vi "svx_Orbit Manage Grid.vi"(4 "Minor Color":u32, 6 "Major Color":u32, 7 "Axis":enum16{"X-Scale", "Y-Scale", "Z-Scale"}(ring), 10 "Grid Style":u16, 11 "Orbit Plot":refnum<vi>) -> (1 "Minor Disabled":u8, 2 "Major Disabled":u8, 3 "Orbit Plot out":refnum<vi>)   [LabVIEW 2017, in "SVX Orbit.xctl"]
uses:
  <vilib>/addons/_XControls/Orbit Plot/SVX Orbit.xctl
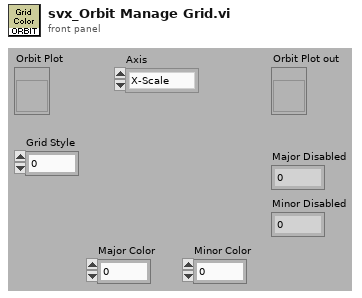
[diagram p1: front panel]
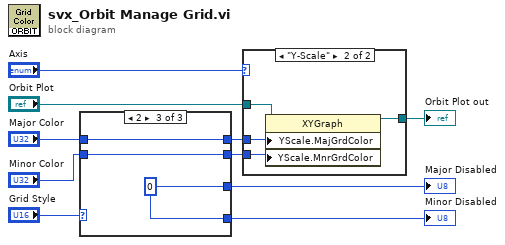
[diagram p0: block diagram]
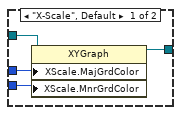
[diagram p2: hidden frame]
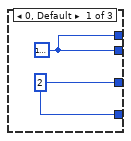
[diagram p3: hidden frame]
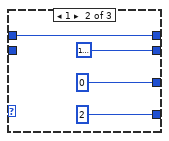
[diagram p4: hidden frame]
diagram:
  n1 = case shown="2" "Grid Style" {
    tunnel: [w12 u8 0 ("Disabled") w19] -> w7
    tunnel: [w12 u8 2 ("Disabled") w19] -> w6
    tunnel: [w11 w13 w18] -> w10
    tunnel: [w11 u32 16777216 w17] -> w5
    tunnel: "Major Color" -> [_ w13 w18]
    tunnel: "Minor Color" -> [_ _ w17]
    frame 0, Default {
      w11 = u32 16777216
      w12 = u8 2 ("Disabled")
    }
    frame 1 {
    }
    frame 2 {
      w19 = u8 0 ("Disabled")
    }
  }
  "Major Disabled" <- w7
  "Minor Disabled" <- w6
  n2 = case shown="\"Y-Scale\"" "Axis" {
    tunnel: w10 -> [w23 w27]
    tunnel: "Orbit Plot" -> [w22 w26]
    tunnel: w5 -> [w21 w25]
    tunnel: [w20 w24] -> w1
    frame "X-Scale", Default {
      n3 = property class="XYGraph"(reference=w22, "XScale.MajGrdColor"=w23, "XScale.MnrGrdColor"=w21) -> (reference out=w20:refnum<vi>)  [unwired: 1 in, 1 out]
    }
    frame "Y-Scale" {
      n4 = property class="XYGraph"(reference=w26, "YScale.MajGrdColor"=w27, "YScale.MnrGrdColor"=w25) -> (reference out=w24:refnum<vi>)  [unwired: 1 in, 1 out]
    }
  }
  "Orbit Plot out" <- w1
